vi "GetAmplitude(V).vi"(0 "object in":refnum<class "AD2_WFG_SDK.lvclass">, 5 "error in (no error)":errorcluster) -> (14 "object out":refnum<class "AD2_WFG_SDK.lvclass">, 16 "Config.Ch1.Carrier.Amplitude (V)":dbl, 17 "Config.Ch2.Carrier.Amplitude (V)":dbl, 19 "error out":errorcluster)   [LabVIEW 2019, in "AD2_WFG_SDK.lvclass"]
uses:
  AD2_WFG_SDK.lvclass
  AD2_WFG_SDK.lvclass/AD2_WFG_SDK.ctl
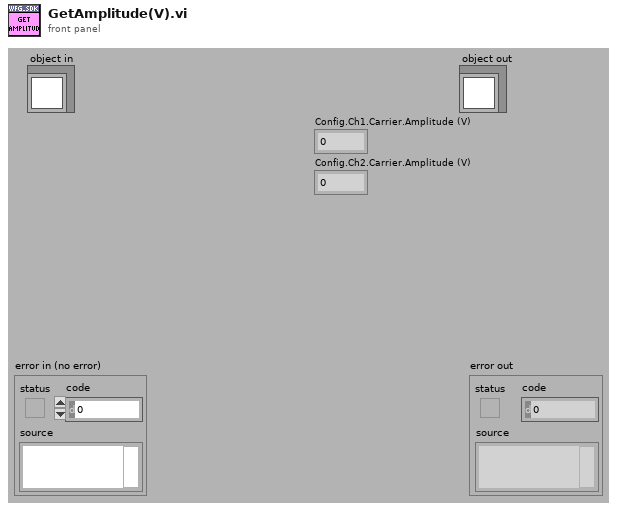
[diagram p1: front panel]
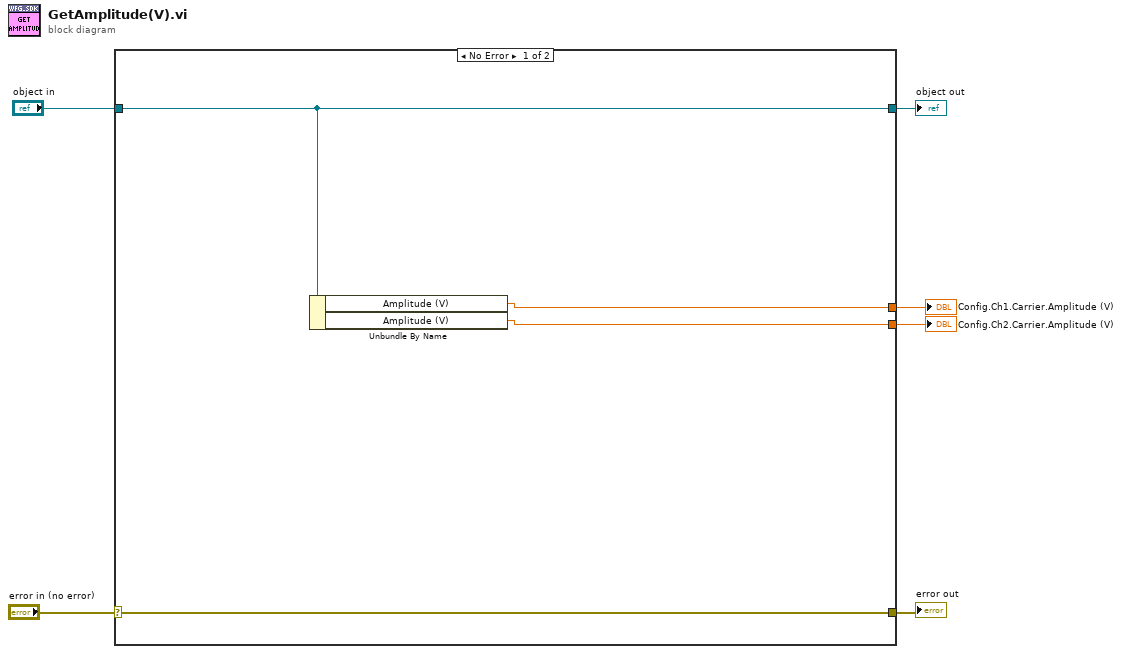
[diagram p0: block diagram]
diagram:
  n1 = case shown="No Error" "error in (no error)" {
    selector: "error in (no error)" -> [w10 w12]
    tunnel: [w10 w12] -> w5
    tunnel: [w9 w11] -> w3
    tunnel: "object in" -> [w9 w11]
    tunnel: [w8 _] -> w2
    tunnel: [w7 _] -> w1
    frame No Error {
      n2 = Unbundle By Name(w9) -> ("Amplitude (V)"=w7:dbl, "Amplitude (V)"=w8:dbl)
    }
    frame Error {
    }
  }
  "error out" <- w5
  "object out" <- w3
  "Config.Ch1.Carrier.Amplitude (V)" <- w1
  "Config.Ch2.Carrier.Amplitude (V)" <- w2
